vi "Power Fit.vi"(9 "parameter bounds":T1, 10 "Integration Times":dbl[](array[numeric]), 11 "Slopes":dbl[](array[numeric])) -> (2 "Power Model":dbl[](array[numeric]), 3 "Fit Verification":cluster{dbl[], "Best Power Fit":dbl[]}[](array[cluster]))   [LabVIEW 2014, in "AvaSpec.lvlib" / "Dark.lvlib"]
uses:
  Dark.lvlib
  <vilib>/Analysis/NI_AALPro.lvlib
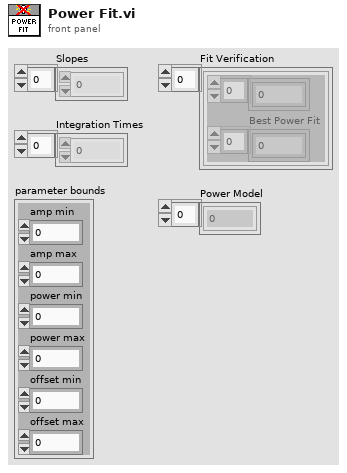
[diagram p1: front panel]
types:
  T1 = cluster{"amp min":dbl, "amp max":dbl, "power min":dbl, "power max":dbl, "offset min":dbl, "offset max":dbl}
  T2 = cluster{"Integration Times":dbl[], "Slopes":dbl[]}
  T3 = cluster{"Integration Times":dbl[], "Best Power Fit":dbl[]}
  T4 = cluster{"Integration Times":dbl[], "Best Power Fit":dbl[]}[]
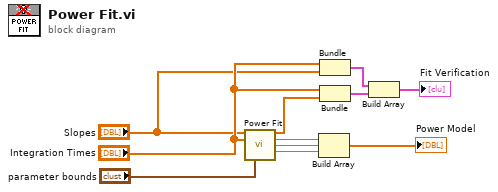
[diagram p0: block diagram]
diagram:
  n1 = call <vilib>:"Power Fit.vi"("Y"="Slopes", "X"="Integration Times", "parameter bounds"="parameter bounds") -> ("Best Power Fit"=w6:dbl[], "amplitude"=w1:dbl, "power"=w2:dbl, "offset"=w3:dbl)  [unwired: 7 in, 2 out]
  n2 = Build Array(w1, w2, w3) -> (→"Power Model":dbl[])
  n3 = Bundle("Integration Times"="Integration Times", "Slopes"="Slopes") -> (w7:T2)  [unwired: 1 in]
  n4 = Bundle("Integration Times"="Integration Times", "Best Power Fit"=w6) -> (w8:T3)  [unwired: 1 in]
  n5 = Build Array(w7, w8) -> (→"Fit Verification":T4)
